vi "AnguloLimite2V2.vi"(6 "XdoAttacker":dbl, 8 "atacando contra":bool, 9 "AnguloAttacker":dbl, 10 "IA State":T1={"our_robots"=[], "enemy_robots"=[], "balls"=[], "geometry"={"line_width"=0, "field_length"=0, "field_width"=0, "boundary_width"=0, "referee_width"=0, "goal_width"=0, "goal_depth"=0, "goal_wall_width"=0, "center_circle_radius"=0, "defense_radius"=0, "defense_stretch"=0, "free_kick_from_defense_dist"=0, "penalty_spot_from_field_line_dist"=0, "penalty_line_from_spot_dist"=0}, "IA Judge"={"stage"="", "command"="", "our_goalie_id"=0.0, "enemy_goalie_id"=0.0, "command enum"=enum."Halt", "Time"=enum."Azul"}, "Received Timestamp"=timestamp(0 s since 1904-01-01), "Events"={"Touch"=FALSE, "Ball out"=FALSE, "id touch"=0.0, "Ball out of \nVision"=FALSE, "Ball inside \nGoalie area"=FALSE, "Robot not responding"=FALSE, "Robots responding status"=[1.0, 1.0, 1.0, 1.0, 1.0, 1.0], "Enemy Ball \nPossession"=FALSE, "Pass State"=FALSE, "id end of pass"=0.0, "Kick"=FALSE, "Id ini Possession"=0.0, "Ball Possesion"=FALSE, "Id Possesion"=0.0, "Direct Kick"=FALSE, "2nd Strk Ativo"=FALSE}}, 11 "YdoAttacker":dbl) -> (1 "Angulo Limite":dbl)   [LabVIEW 2017]
uses:
  Core/AI Input.ctl
  Core/AI Robot.ctl
  Intel/Functions Enum.ctl
  Intel/AttackerStates.ctl
  Path Planning/RRT/PathDests.ctl
  Path Planning/RRT/PathDest.ctl
  Core/AI Ball.ctl
  Core/Field Size.ctl
  Core/AI Judge.ctl
  Intel/Command Enum.ctl
  Events/Events.ctl
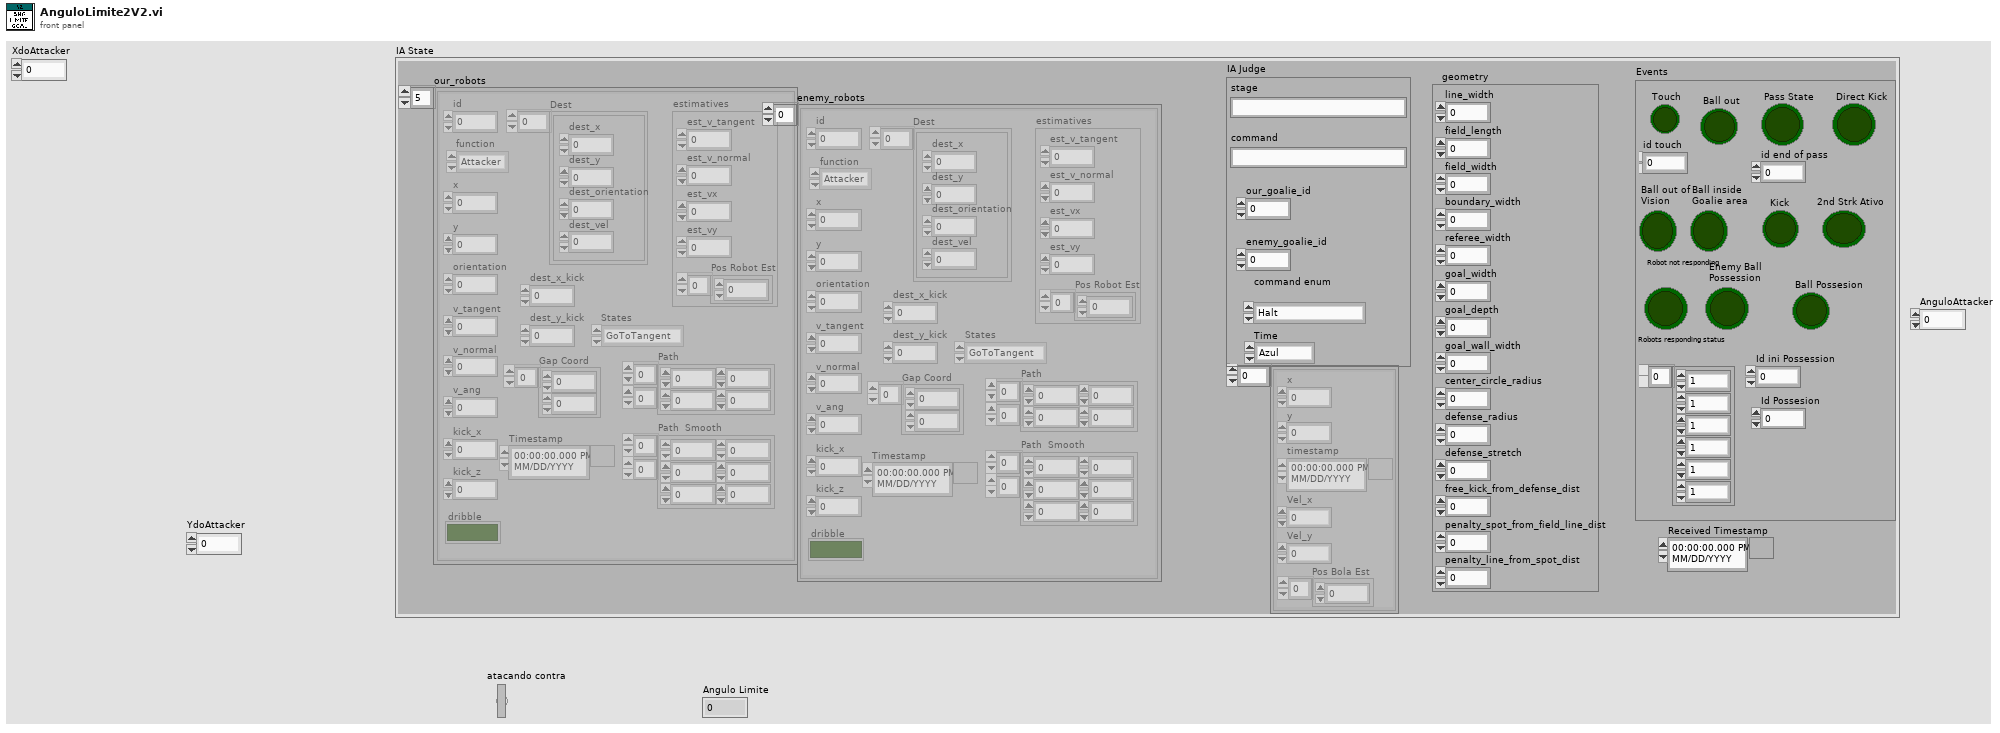
[diagram p1: front panel]
types:
  T1 = typedef "AI Input.ctl" = cluster{"our_robots":T2[], "enemy_robots":T2[], "balls":T7[], "geometry":T8, "IA Judge":T9, "Received Timestamp":timestamp, "Events":T11}
  T2 = typedef "AI Robot.ctl" = cluster{"id":u32, "function":T3, "x":dbl, "y":dbl, "orientation":dbl, "v_tangent":dbl, "v_normal":dbl, "v_ang":dbl, "kick_x":dbl, "kick_z":dbl, "dribble":bool, "Timestamp":timestamp, "estimatives":cluster{"est_v_tangent":dbl, "est_v_normal":dbl, "est_vx":dbl, "est_vy":dbl, "Pos Robot Est":dbl[]}, "dest_x_kick":dbl, "dest_y_kick":dbl, "Gap Coord":dbl[], "States":T4, "Path ":dbl[][], "Path  Smooth":dbl[][], "Dest":T5}
  T3 = typedef "Functions Enum.ctl" = enum16{"2nd Striker", "Attacker", "Goalie", "Defender", "Striker", "Goto 0", "Dummy", "Kicker", "ZigZag 0", "ZigZag 1", "ZigZag 2", "ZigZag 3", "ZigZag 4", "ZigZag 5", "ZigZag 6", "ZigZag 7", "ZigZag 8", ""}
  T4 = typedef "AttackerStates.ctl" = enum16{"Pass", "GoToTangent", "BallGetting", "GoToKick", ""}
  T5 = typedef "PathDests.ctl" = T6[]
  T6 = typedef "PathDest.ctl" = cluster{"dest_x":dbl, "dest_y":dbl, "dest_orientation":dbl, "dest_vel":dbl}
  T7 = typedef "AI Ball.ctl" = cluster{"x":dbl, "y":dbl, "timestamp":timestamp, "Vel_x":dbl, "Vel_y":dbl, "Pos Bola Est":dbl[]}
  T8 = typedef "Field Size.ctl" = cluster{"line_width":u32, "field_length":u32, "field_width":u32, "boundary_width":u32, "referee_width":u32, "goal_width":u32, "goal_depth":u32, "goal_wall_width":u32, "center_circle_radius":u32, "defense_radius":u32, "defense_stretch":u32, "free_kick_from_defense_dist":u32, "penalty_spot_from_field_line_dist":u32, "penalty_line_from_spot_dist":u32}
  T9 = typedef "AI Judge.ctl" = cluster{"stage":string, "command":string, "our_goalie_id":dbl, "enemy_goalie_id":dbl, "command enum":T10, "Time":enum16{"Azul", "Amarelo"}}
  T10 = typedef "Command Enum.ctl" = enum16{"Halt", "Stop", "Force Start", "PKA Normal Start", "Prepare Kickoff Ally", "PKE Normal Start", "Prepare Kickoff Enemy", "Prepare Penalty Ally", "PPA Normal Start", "Prepare Penalty Enemy", "PPE Normal Start", "Direct Free Enemy", "Direct Free Ally", "Indirect Free Enemy", "Indirect Free Ally", "Timeout Enemy", "Timeout Ally", "Goal Enemy", "Goal Ally", "Ball Placement Enemy", "Ball Placement Ally", "Normal Half Time", "Extra Time Break", "Extra Half Time", "None", "Post Game"}
  T11 = typedef "Events.ctl" = cluster{"Touch":bool, "Ball out":bool, "id touch":dbl, "Ball out of \nVision":bool, "Ball inside \nGoalie area":bool, "Robot not responding":bool, "Robots responding status":dbl[], "Enemy Ball \nPossession":bool, "Pass State":bool, "id end of pass":dbl, "Kick":bool, "Id ini Possession":dbl, "Ball Possesion":bool, "Id Possesion":dbl, "Direct Kick":bool, "2nd Strk Ativo":bool}
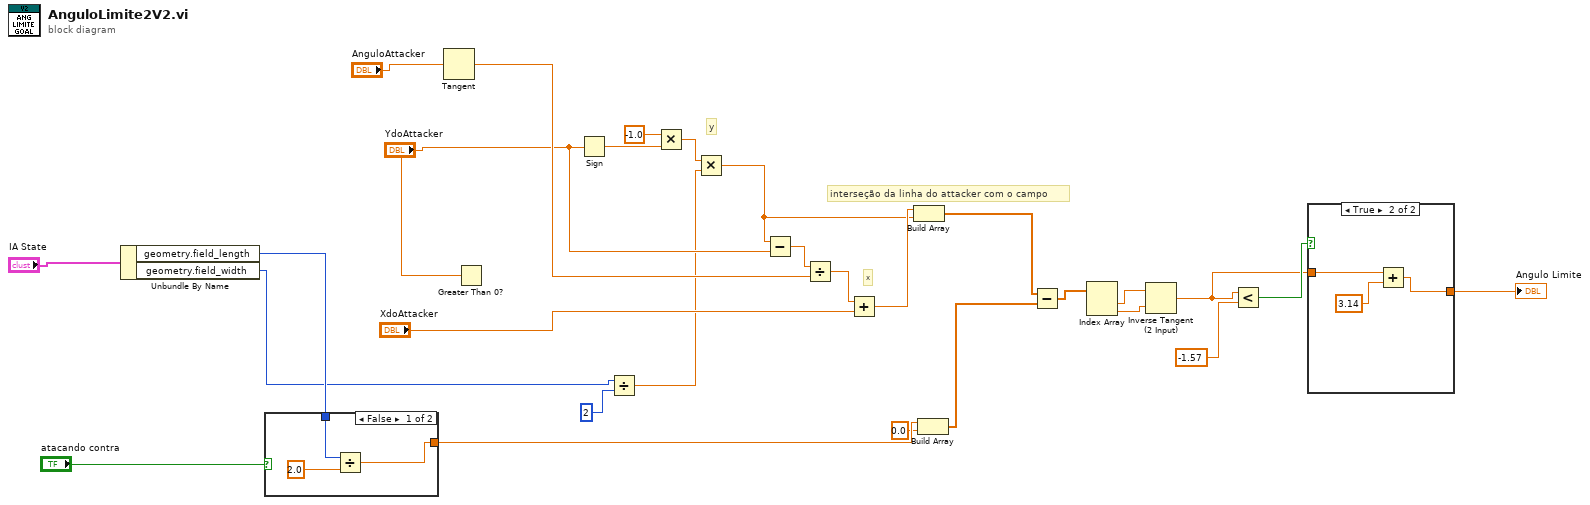
[diagram p0: block diagram]
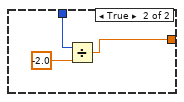
[diagram p3: hidden frame]
diagram:
  # "interseção da linha do attacker com o campo"
  # "x"
  # "y"
  n1 = Unbundle By Name("IA State") -> ("geometry.field_length"=w27:u32, "geometry.field_width"=w26:u32)
  n2 = case shown="False" "atacando contra" {
    tunnel: w27 -> [w30 w34]
    tunnel: [w29 w32] -> w8
    frame False {
      n3 = Divide(x=w30, y=2.0) -> (x/y=w29:dbl)
    }
    frame True {
      n4 = Divide(x=w34, y=-2.0) -> (x/y=w32:dbl)
    }
  }
  n5 = Tangent(1:"AnguloAttacker") -> (0:w24:dbl)
  n6 = Greater Than 0?(x="YdoAttacker") -> ()  [unwired: 1 out]
  n7 = Sign(1:"YdoAttacker") -> (0:w20:dbl)
  n8 = Divide(x=w26, y=u32 2) -> (x/y=w16:dbl)
  n9 = Multiply(x=-1.0, y=w20) -> (x*y=w17:dbl)
  n10 = Multiply(x=w17, y=w16) -> (x*y=w12:dbl)
  n11 = Subtract(x=w12, y="YdoAttacker") -> (x-y=w15:dbl)
  n12 = Divide(x=w15, y=w24) -> (x/y=w14:dbl)
  n13 = Add(x=w14, y="XdoAttacker") -> (x+y=w13:dbl)
  n14 = Build Array(w13, w12) -> (w11:dbl[])
  n15 = Build Array(w8, 0.0 ("element")) -> (w10:dbl[])
  n16 = Subtract(x=w11, y=w10) -> (x-y=w9:dbl[])
  n17 = Index Array(array=w9) -> (element #1=w2:dbl, element #2=w1:dbl)  [unwired: 2 in]
  n18 = Inverse Tangent (2 Input)(1:w1, 2:w2) -> (0:w4:dbl)
  n19 = Less?(x=w4, y=-1.57) -> (x < y?=w5:bool)
  n20 = case shown="True" w5 {
    tunnel: w4 -> [w35 w38]
    tunnel: [w35 w36] -> w3
    frame False {
    }
    frame True {
      n21 = Add(x=w38, y=3.14) -> (x+y=w36:dbl)
    }
  }
  "Angulo Limite" <- w3
